vi "niFPGA BW CU Order 2  n-chan (16-bit).vi"(0 "filter state in":i32[](array[numeric])=[0, 0, 0], 1 "reset":bool, 5 "input data":i16, 7 "accumulator in":i32, 9 "adder in":i32, 11 "iteration":u8, 13 "lowpass?":bool) -> (4 "filter state out":i32, 6 "state to multiply":i32, 8 "accumulator out":i32, 10 "adder out":i32, 15 "terminate":bool)   [LabVIEW 2017]
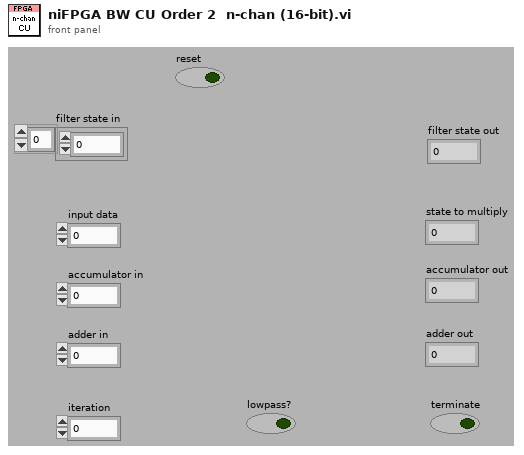
[diagram p1: front panel]
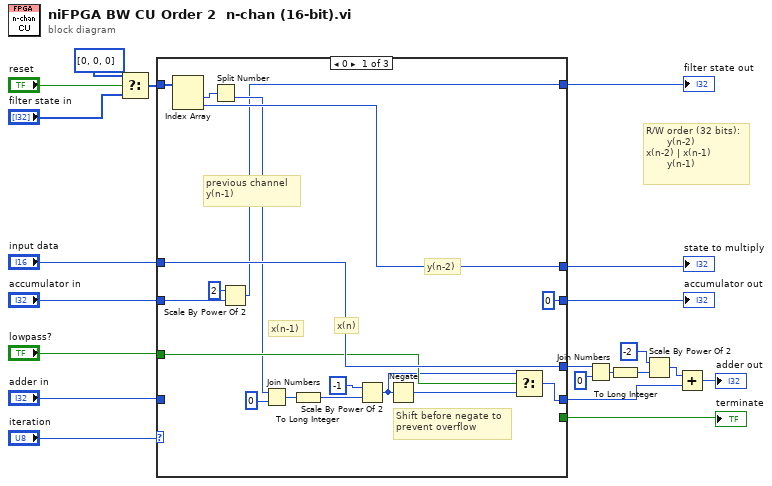
[diagram p0: block diagram]
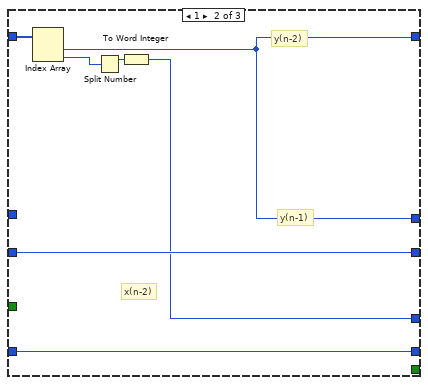
[diagram p2: hidden frame]
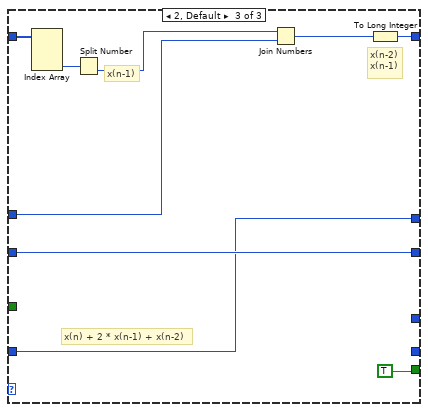
[diagram p3: hidden frame]
diagram:
  # "R/W order (32 bits):\n       y(n-2)\nx(n-2) | x(n-1)\n       y(n-1)"
  n1 = Select(t=i32[] [0, 0, 0], s="reset", f="filter state in") -> (s? t:f=w10:i32[])
  n2 = case shown="0" "iteration" {
    tunnel: "input data" -> [w31 _ w51]
    tunnel: [w23 w45 _] -> w21
    tunnel: "adder in" -> [_ w45 w53]
    tunnel: [w29 w40 w53] -> w15
    tunnel: [w31 w39 _] -> w4
    tunnel: "accumulator in" -> [w37 w44 w54]
    tunnel: [0 ("Numeric") w44 w54] -> w14
    tunnel: [_ _ TRUE] -> w19
    tunnel: [w26 w40 w46] -> w2
    tunnel: w10 -> [w35 w43 w49]
    tunnel: "lowpass?" -> [w30 _ _]
    frame 0 {
      # "Shift before negate to\nprevent overflow"
      # "previous channel \ny(n-1)"
      # "x(n)"
      # "x(n-1)"
      # "y(n-2)"
      n3 = Index Array(array=w35) -> (element #1=w28:i32, element #2=w29:i32)  [unwired: 2 in]
      n4 = Split Number(x=w28) -> (lo(x)=w27:u16)  [unwired: 1 out]
      n5 = Scale By Power Of 2(n=2, x=w37) -> (x*2^n=w26:i32)
      n6 = Join Numbers(hi=w27, lo=i16 0) -> ((hi.lo)=w34:u32)
      n7 = To Long Integer(number=w34) -> (32bit integer=w25:i32)
      n8 = Scale By Power Of 2(n=-1, x=w25) -> (x*2^n=w24:i32)
      n9 = Negate(x=w24) -> (-x=w32:i32)
      n10 = Select(t=w24, s=w30, f=w32) -> (s? t:f=w23:i32)
    }
    frame 1 {
      # "y(n-2)"
      # "x(n-2)"
      # "y(n-1)"
      n11 = Index Array(array=w43) -> (element #1=w40:i32, element #2=w42:i32)  [unwired: 2 in]
      n12 = Split Number(x=w42) -> (hi(x)=w41:u16)  [unwired: 1 out]
      n13 = To Word Integer(number=w41) -> (16bit integer=w39:i16)
    }
    frame 2, Default {
      # "x(n-1)"
      # "x(n-2)\nx(n-1)"
      # "x(n) + 2 * x(n-1) + x(n-2)"
      n14 = Index Array(array=w49) -> (element #3=w48:i32)  [unwired: 3 in, 2 out]
      n15 = Split Number(x=w48) -> (lo(x)=w47:u16)  [unwired: 1 out]
      n16 = Join Numbers(hi=w47, lo=w51) -> ((hi.lo)=w50:u32)
      n17 = To Long Integer(number=w50) -> (32bit integer=w46:i32)
    }
  }
  "state to multiply" <- w15
  "terminate" <- w19
  "accumulator out" <- w14
  "filter state out" <- w2
  n18 = Join Numbers(hi=w4, lo=i16 0) -> ((hi.lo)=w7:u32)
  n19 = To Long Integer(number=w7) -> (32bit integer=w6:i32)
  n20 = Scale By Power Of 2(n=-2, x=w6) -> (x*2^n=w3:i32)
  n21 = Add(x=w3, y=w21) -> (x+y=→"adder out":i32)
